vi "删除数组元素.vi"() -> ()   [LabVIEW 2012]
panel:
  out "已删除的部分":i32[](array[numeric])
  out "已删除元素的数组子集":i32[](array[numeric])
  out "已删除的部分2":i32[](array[numeric])
  out "已删除元素的数组子集2":i32[](array[numeric])
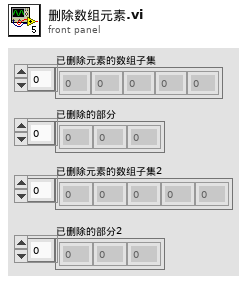
[diagram p1: front panel]
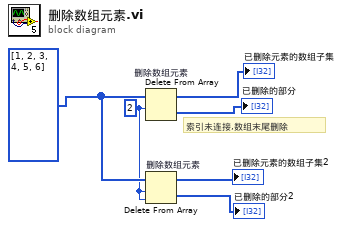
[diagram p0: block diagram]
diagram:
  w5 = 2 ("长度")
  w6 = i32[] [1, 2, 3, 4, 5, 6]
  # "索引未连接,数组末尾删除"
  n1 = Delete From Array "删除数组元素"(array=w6, length=w5) -> (deleted portion=→"已删除的部分":i32[], array with subset deleted=→"已删除元素的数组子集":i32[])  [unwired: 1 in]
  n2 = Delete From Array "删除数组元素"(array=w6, length=w5, index=w5) -> (deleted portion=→"已删除的部分2":i32[], array with subset deleted=→"已删除元素的数组子集2":i32[])
